vi "Column Widths Write.vi"(4 "error in (no error)":errorcluster, 5 "Value":i32[](array[numeric]), 6 "Container State":T3, 7 "Display State In":T1={"logTable"=refnum, "max items"=500, "displaydata"=[], "data"=[], "Auto Scroll"=TRUE, "current item"=500, "col headers"=[], "Add to Top"=TRUE, "Auto resize"=TRUE, "col size"=[], "filters"=[], "color cells"=[]}) -> (0 "error out":errorcluster, 3 "Display State Out":T1={"logTable"=refnum, "max items"=500, "displaydata"=[], "data"=[], "Auto Scroll"=TRUE, "current item"=500, "col headers"=[], "Add to Top"=TRUE, "Auto resize"=TRUE, "col size"=[], "filters"=[], "color cells"=[]})   [LabVIEW 2017, in "UI-DisplayTable(dev).xctl"]
uses:
  UI-DisplayTable(dev).xctl
  <vilib>/_xctls/Container State.ctl
  State.ctl
  Support/DEF-Filter.ctl
  <vilib>/_xctls/XControlSupport.lvlib
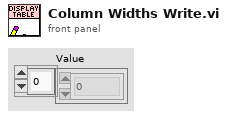
[diagram p1: front panel]
types:
  T1 = typedef "UI-DisplayTable(dev).xctl/State.ctl" = cluster{"logTable":refnum<vi>, "max items":i32, "displaydata":string[][], "data":string[][], "Auto Scroll":bool, "current item":i32, "col headers":string[], "Add to Top":bool, "Auto resize":bool, "col size":i32[], "filters":T2[], "color cells":cluster{"color cell":cluster{"Column":string, "Value":string, "Highlight Column":string}, "Color Box":u32}[]}
  T2 = typedef "UI-DisplayTable(dev).xctl/DEF-Filter.ctl" = cluster{"column":string, "value":string[]}
  T3 = typedef "XControlSupport.lvlib/Container State.ctl" = cluster{"Indicator?":bool, "Run Mode?":bool, " Refnum":refnum<vi>}
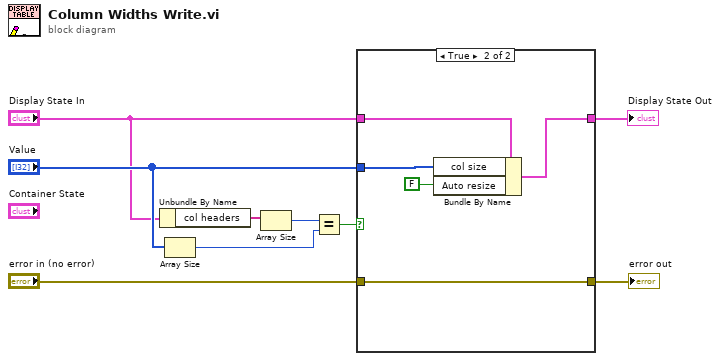
[diagram p0: block diagram]
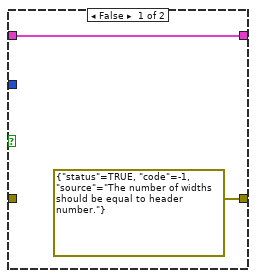
[diagram p2: hidden frame]
diagram:
  n1 = Unbundle By Name("Display State In") -> ("col headers"=w5:string[])
  n2 = Array Size(array="Value") -> (size(s)=w4:i32)
  n3 = Array Size(array=w5) -> (size(s)=w6:i32)
  n4 = Equal?(x=w6, y=w4) -> (x = y?=w3:bool)
  n5 = case shown="True" w3 {
    tunnel: [w11 w16] -> w9
    tunnel: "Value" -> [_ w14]
    tunnel: "Display State In" -> [w11 w13]
    tunnel: "error in (no error)" -> [_ w12]
    tunnel: [errorcluster {"status"=TRUE, "code"=-1, "source"="The number of widths should be equal to header number."} ("error in (no error)") w12] -> w1
    frame False {
    }
    frame True {
      n6 = Bundle By Name(cluster=w13, "col size"=w14, "Auto resize"=FALSE) -> (w16:T1)
    }
  }
  "error out" <- w1
  "Display State Out" <- w9
